vi "measure stable current with transmission.vi"(7 "na/V 2":dbl=1000.0, 8 "error in":errorcluster, 9 "measure ss":bool, 10 "field change wait(s)":u32=5, 11 "na/V":dbl=500.0) -> (0 "error out":errorcluster, 1 "stable current 2":dbl format="%.2f", 3 "stable current":dbl format="%.2f", 4 "inj current":dbl format="%#_6e", 5 "INJ ss ratio":dbl format="%#_6e")   [LabVIEW 2016]
uses:
  stable controls/stable cluster.ctl
  kubley/data acquisition 2009/beamline/controls/stable state combo.ctl
panel:
  in  "Charge State":dbl=3.0
  out "Waveform Graph 2":dbl[](graph)
  in  "measure transmission?":bool=TRUE
  in  "stable data in":T1={"injector current"=1.0, "offset current"=1.0, "ss inj ratio"=1.0, "ss offset ratio"=1.0, "transmission"=1.0, "2nd offset current"=1.0}
  out "stable data out":T1={"injector current"=1.0, "offset current"=1.0, "ss inj ratio"=1.0, "ss offset ratio"=1.0, "transmission"=1.0, "2nd offset current"=1.0}
  out "stable current 3":cluster{"data":dbl[]}[](graph)
  in  "inj current 4":dbl
  out "inj current 3":dbl format="%#_6e"
  in  "inj current 2":dbl
  out "step":string
  in  "measure stable":bool
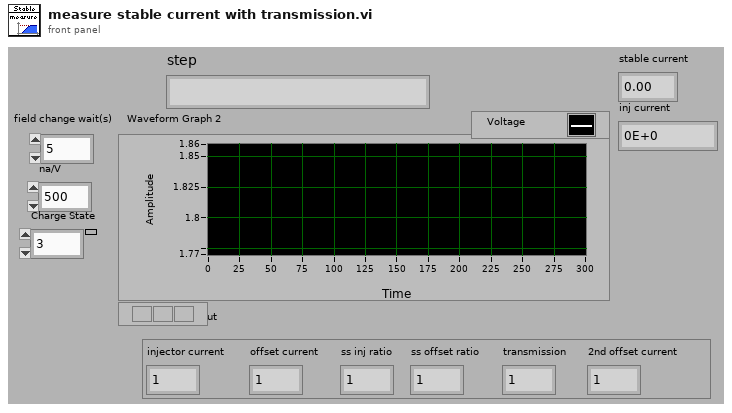
[diagram p1: front panel]
types:
  T1 = typedef "stable cluster.ctl" = cluster{"injector current":dbl, "offset current":dbl, "ss inj ratio":dbl, "ss offset ratio":dbl, "transmission":dbl, "2nd offset current":dbl}
  T2 = typedef "stable state combo.ctl" = string
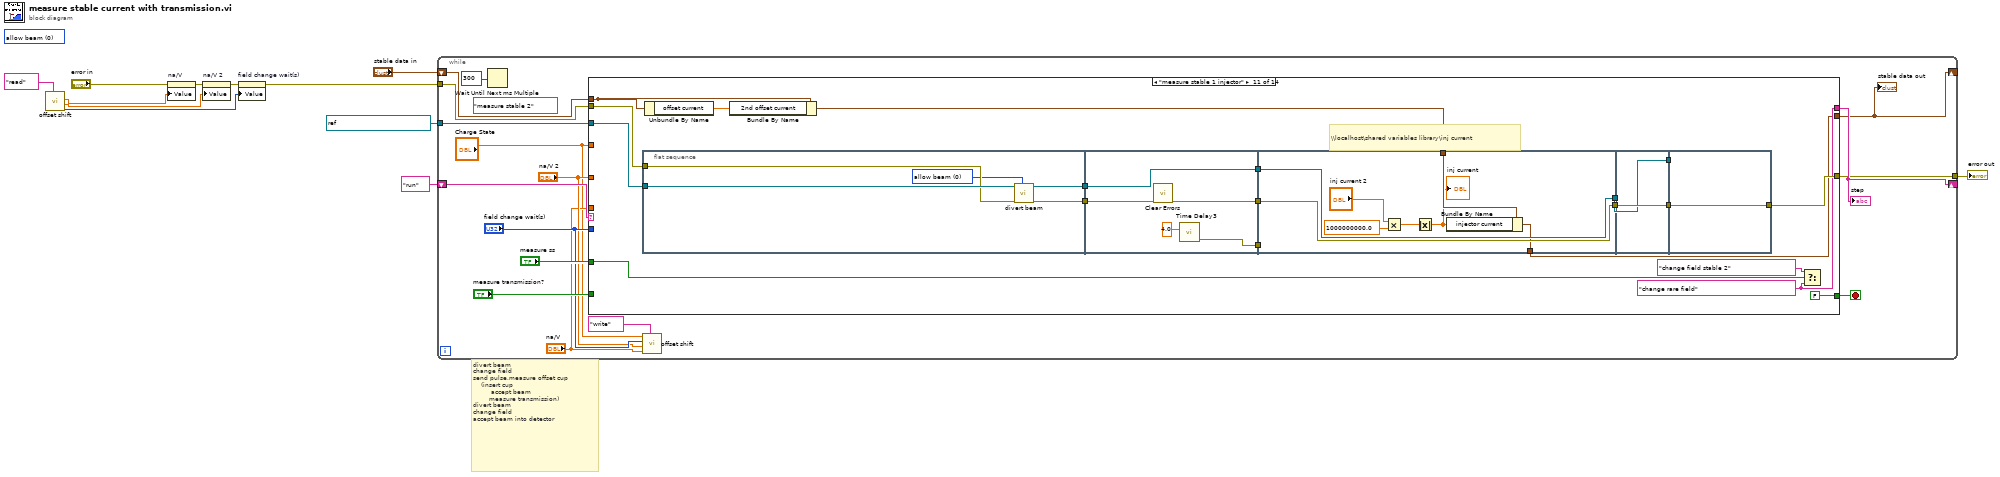
[diagram p0: block diagram]
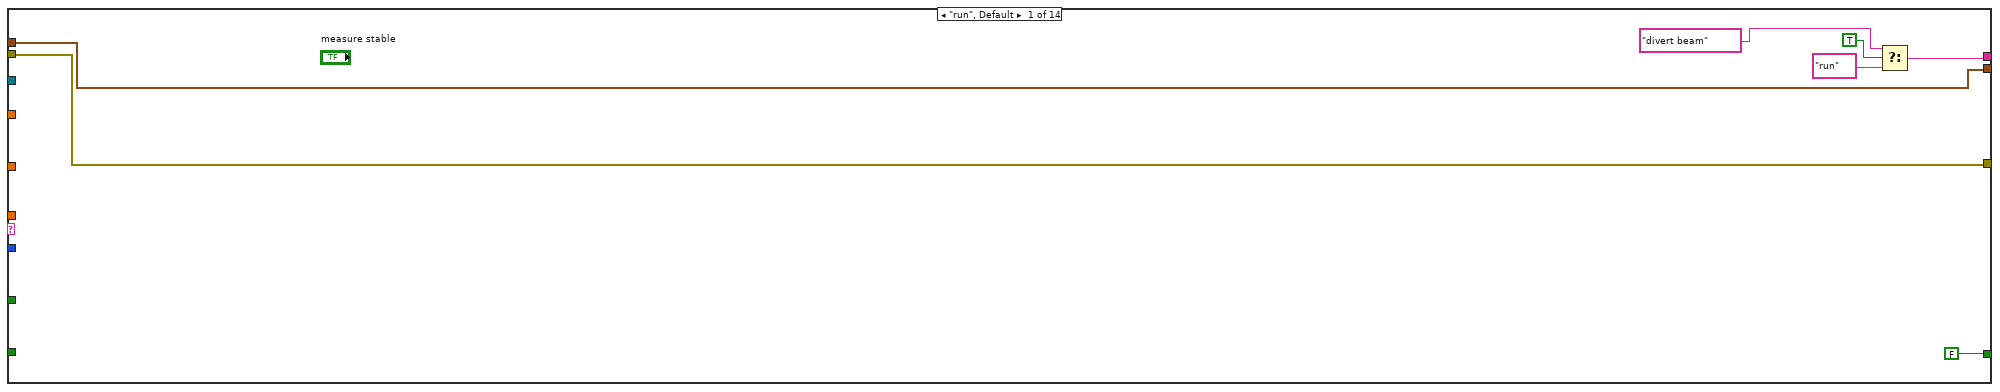
[diagram p2: hidden frame]
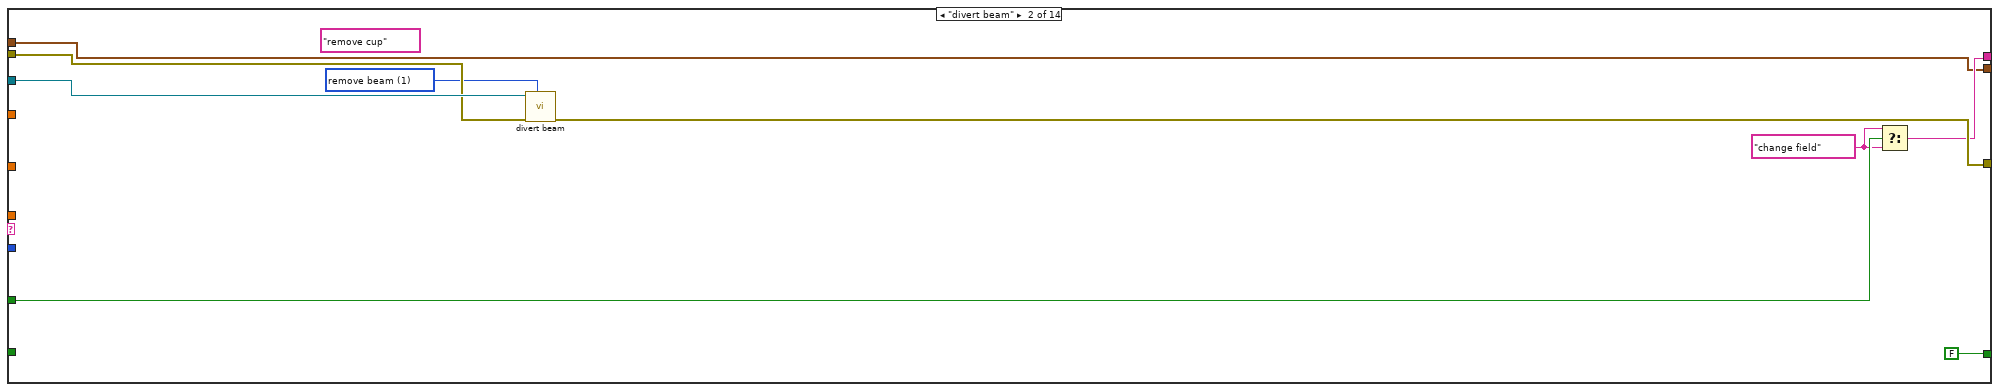
[diagram p3: hidden frame]
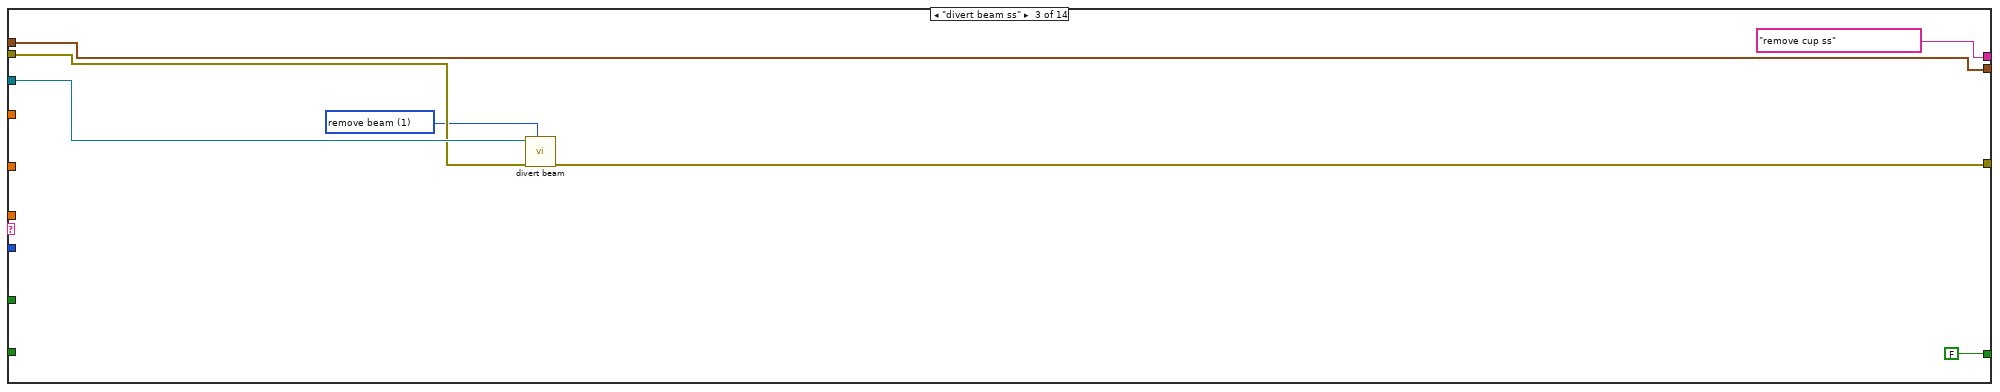
[diagram p4: hidden frame]
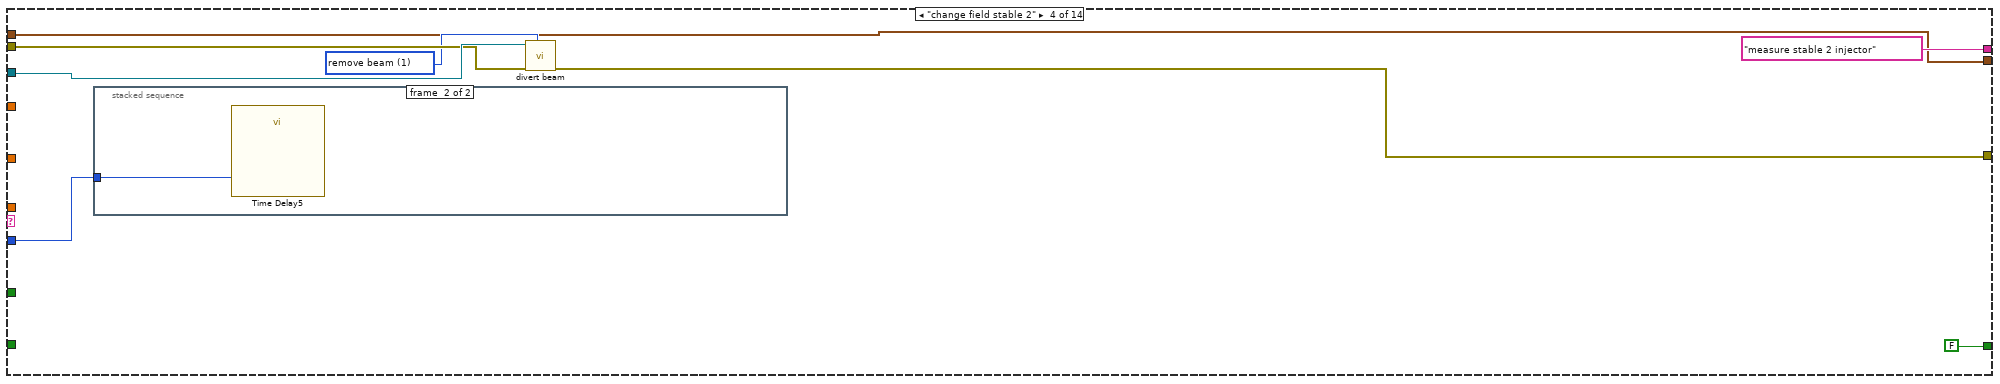
[diagram p5: hidden frame]
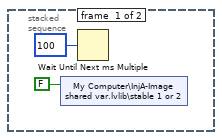
[diagram p6: hidden frame]
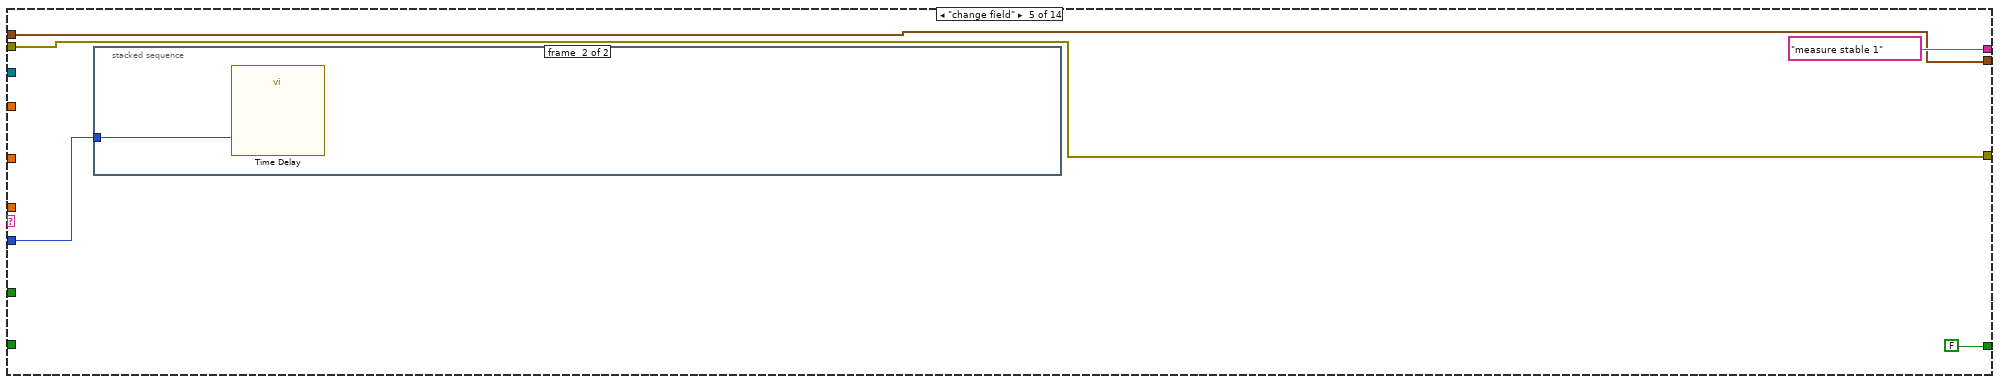
[diagram p7: hidden frame]
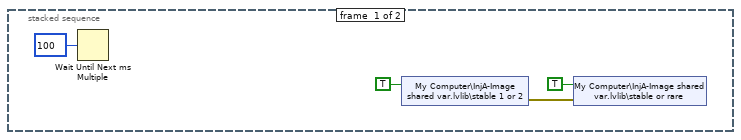
[diagram p8: hidden frame]
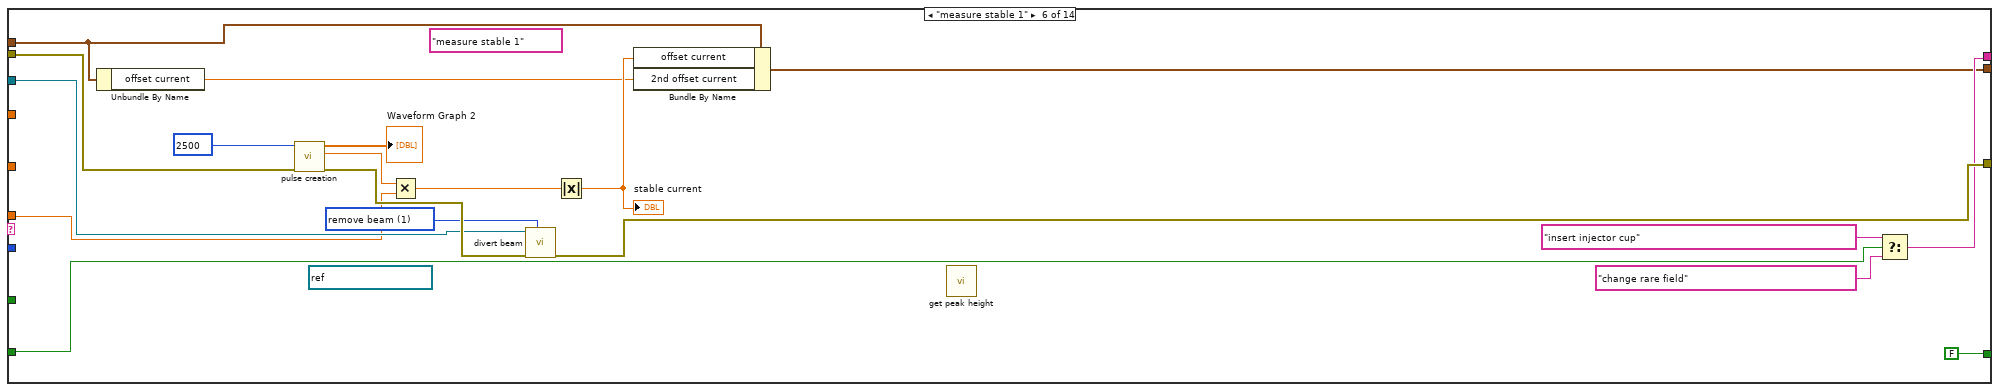
[diagram p9: hidden frame]
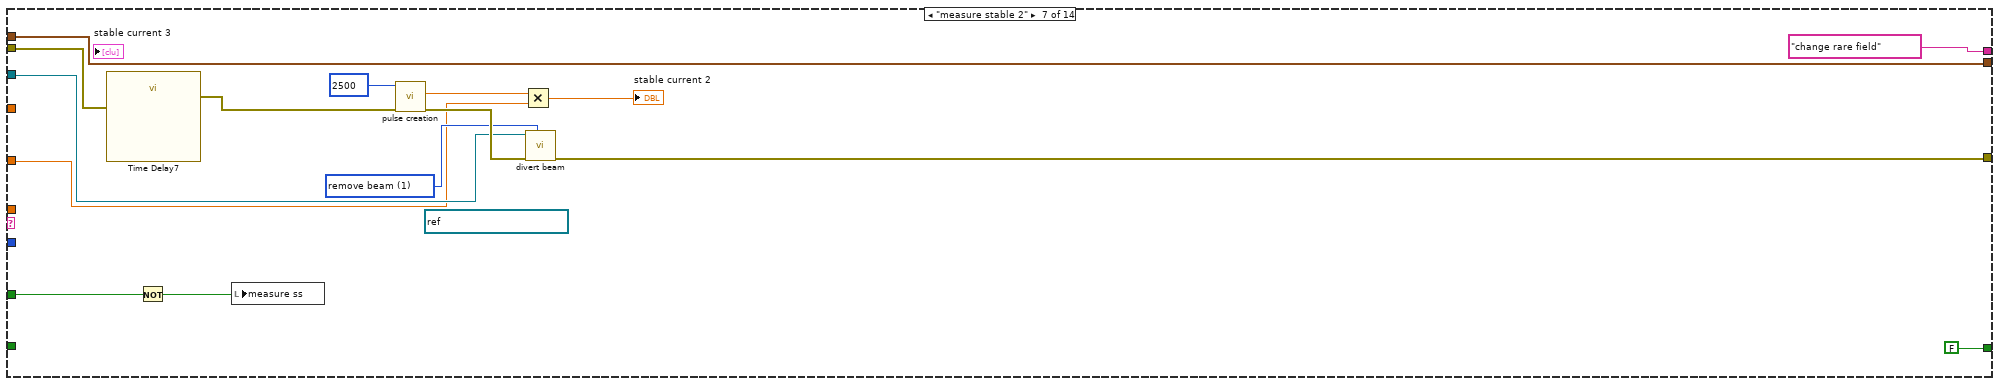
[diagram p10: hidden frame]
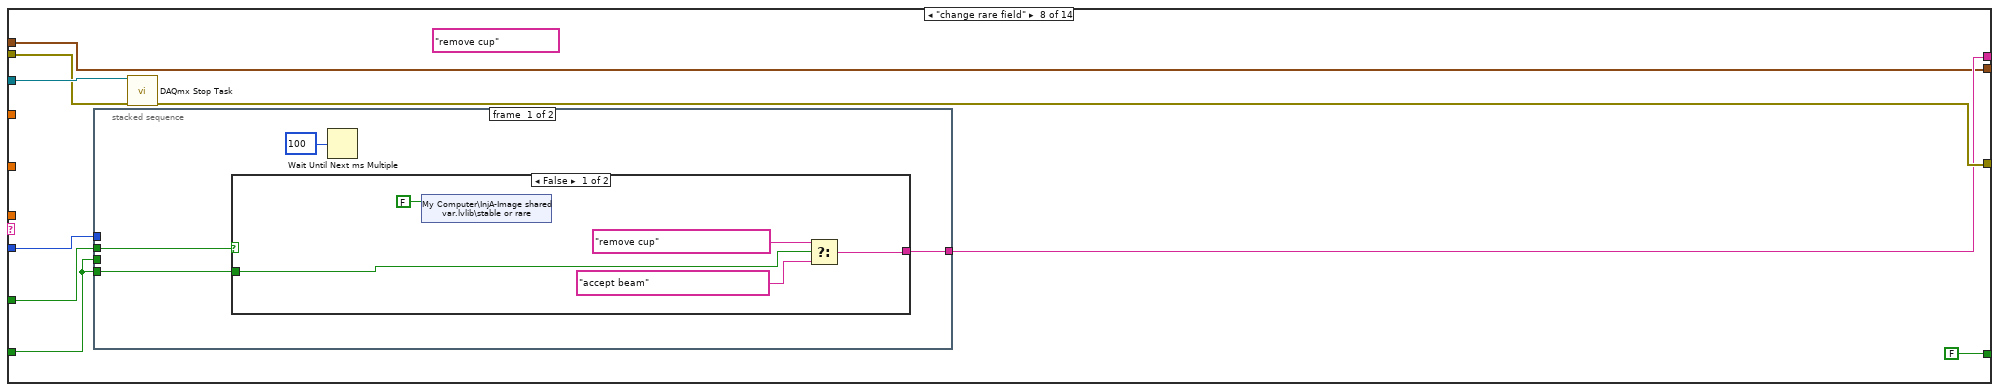
[diagram p11: hidden frame]
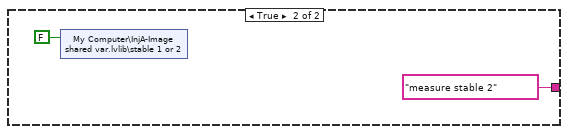
[diagram p12: hidden frame]
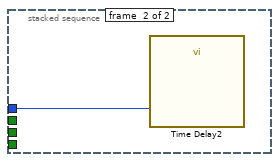
[diagram p13: hidden frame]
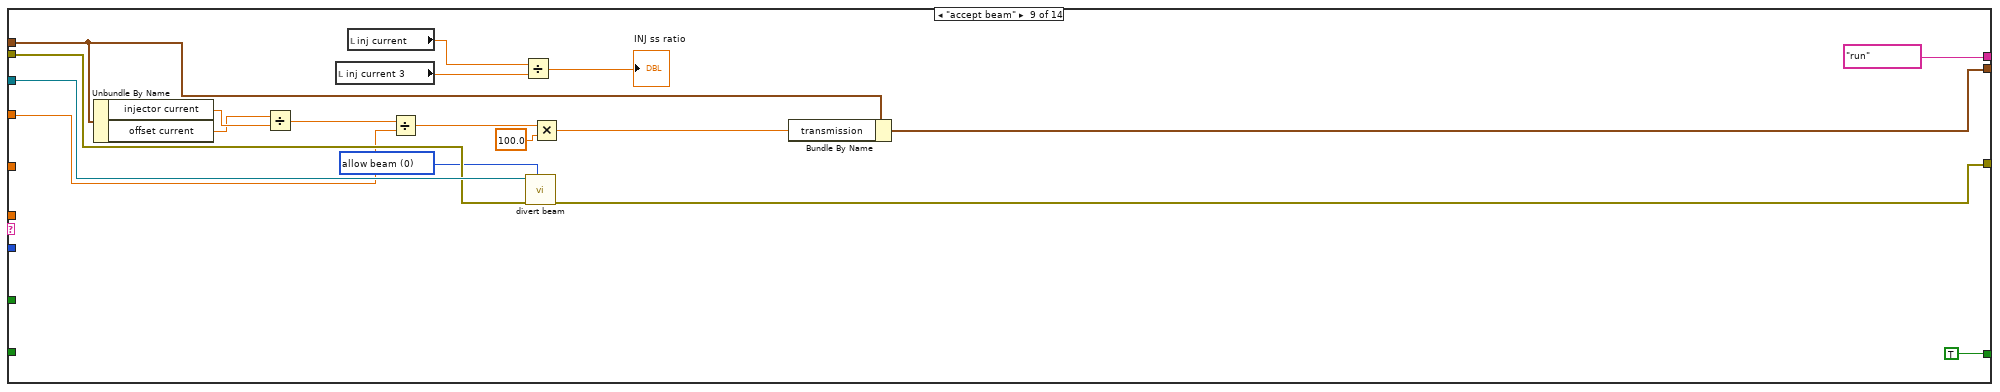
[diagram p14: hidden frame]
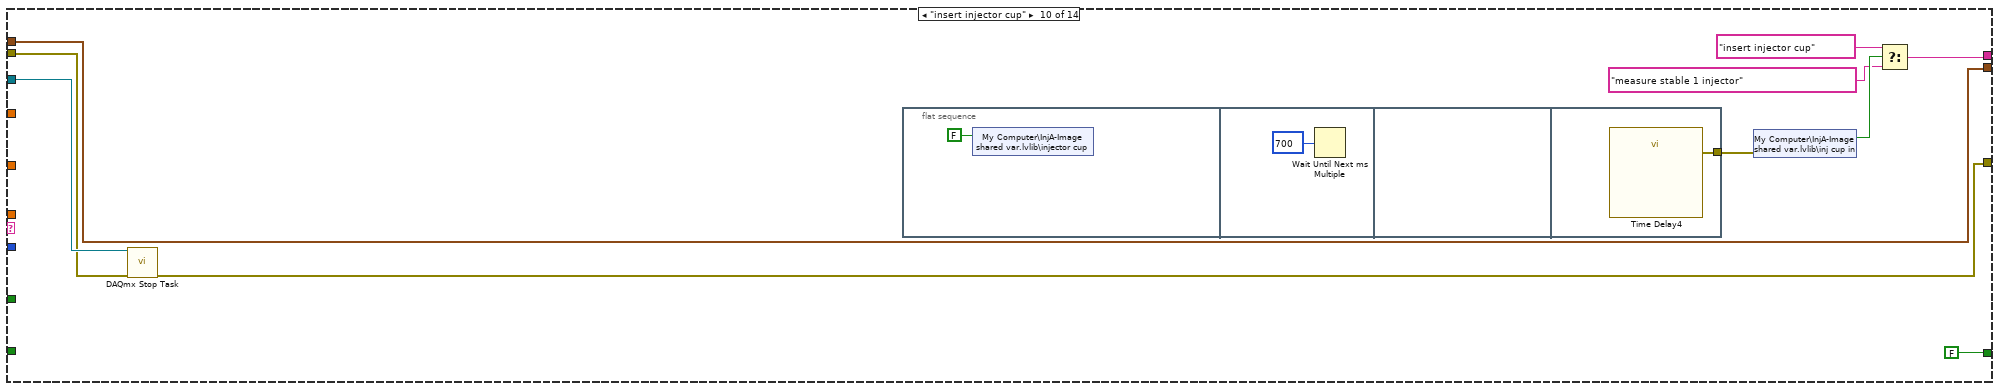
[diagram p15: hidden frame]
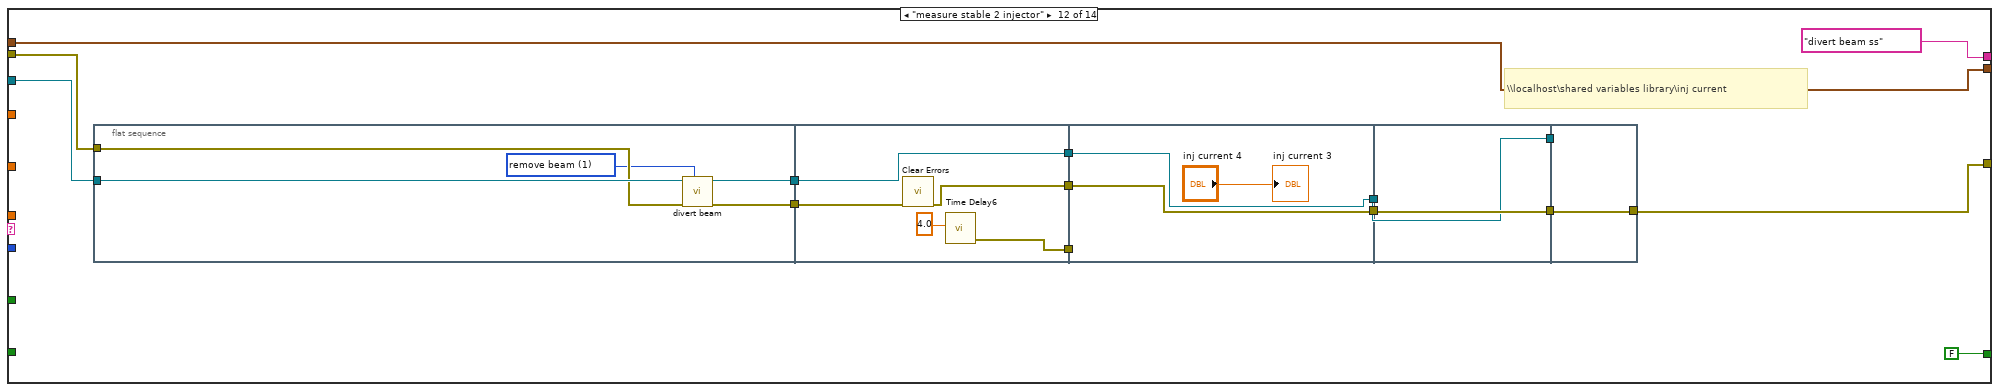
[diagram p16: hidden frame]
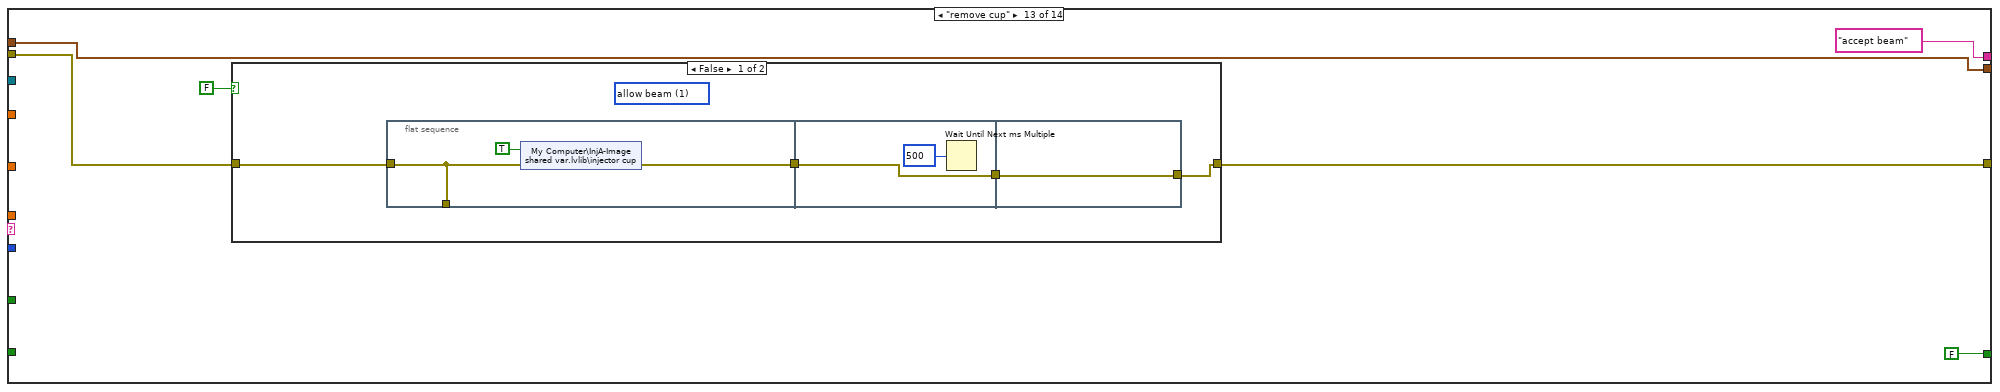
[diagram p17: hidden frame]
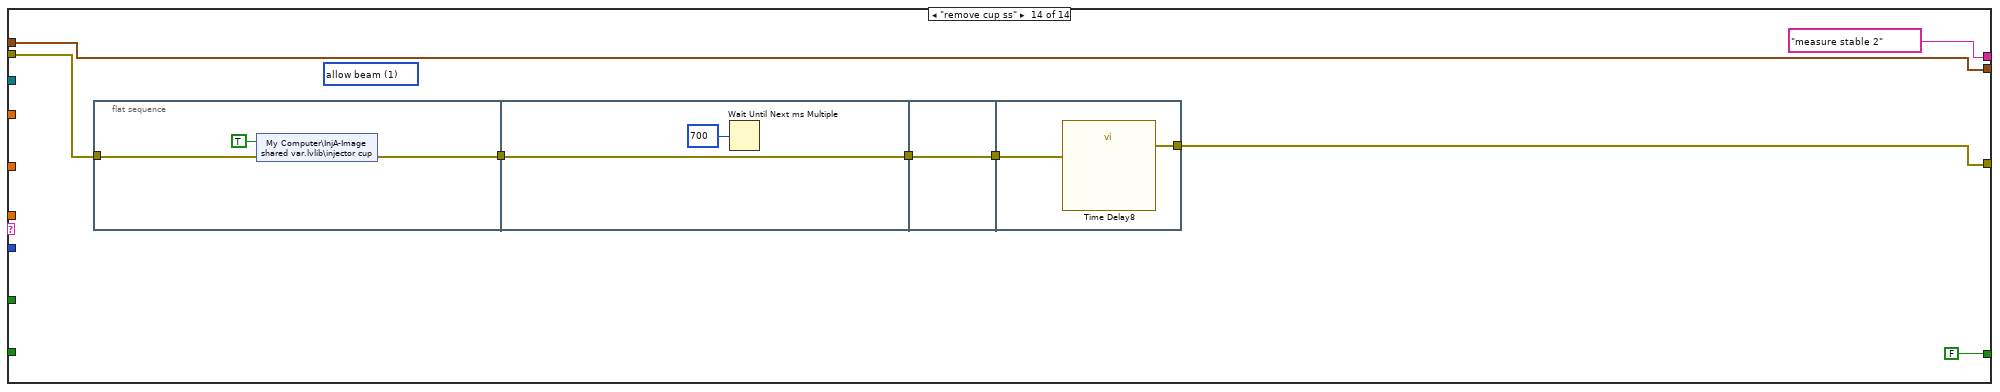
[diagram p19: hidden frame]
diagram:
  (unwired) u16 0 items=["allow beam", "remove beam"] ("divert beam? 2")
  # "divert beam\nchange field\nsend pulse,measure offset cup\n    (insert cup\n         accept beam\n        measure transmission)\ndivert beam\nchange field\naccept beam into detector"
  n1 = call "offset shift.vi"("read writ"="read") -> ("field change wait(s) out"=w8:u32, "na/V 2out"=w7:dbl, "na/V out"=w6:dbl)  [unwired: 7 in, 1 out]
  n2 = property on="na/V" class="DigNum (strict)"(error in="error in", "Value"=w6) -> (error out=w4:errorcluster)  [unwired: 1 in, 1 out]
  n3 = property on="na/V 2" class="DigNum (strict)"(error in=w4, "Value"=w7) -> (error out=w3:errorcluster)  [unwired: 1 in, 1 out]
  n4 = property on="field change wait(s)" class="DigNum (strict)"(error in=w3, "Value"=w8) -> (error out=w2:errorcluster)  [unwired: 1 in, 1 out]
  n5 = while {
    shift-right: [w27] -> _
    shift-left: T2 "run" ("stable measurement type") -> [w28]
    tunnel: refnum<k21> "stable current output" ("task/channels in") -> [w26]
    tunnel: [w24] -> w10
    tunnel: w2 -> [w23]
    shift-right: [w18] -> _
    shift-left: "stable data in" -> [w19]
    stop <- w22 stop-if-true
    (unwired) T2 "measure stable 2" ("stable measurement type")
    n6 = Wait Until Next ms Multiple(millisecond multiple=u32 300) -> ()  [unwired: 1 out]
    n7 = case shown="\"measure stable 1 injector\"" w28 {
      tunnel: [w33 w39 T2 "remove cup ss" ("stable measurement type") T2 "measure stable 2 injector" ("stable measurement type") T2 "measure stable 1" ("stable measurement type") w82 T2 "change rare field" ("stable measurement type") w108 T2 "run" ("stable measurement type") w149 w163 T2 "divert beam ss" ("stable measurement type") T2 "accept beam" ("stable measurement type") T2 "measure stable 2" ("stable measurement type")] -> w27
      tunnel: w26 -> [_ w44 w51 w59 _ w87 w103 w113 w145 w154 w175 w211 _ _]
      tunnel: "field change wait(s)" -> [_ _ _ w54 w66 _ _ w115 _ _ _ _ _ _]
      tunnel: [FALSE ("stop") FALSE ("stop") FALSE ("stop") FALSE ("stop") FALSE ("stop") FALSE ("stop") FALSE ("stop") FALSE ("stop") TRUE ("stop") FALSE ("stop") FALSE ("stop") FALSE ("stop") FALSE ("stop") FALSE ("stop")] -> w22
      tunnel: [w30 w42 w49 w56 w64 w84 w101 w111 w141 w152 w166 w202 w233 w248] -> w24
      tunnel: w23 -> [w30 w41 w48 w55 w64 w88 w97 w112 w142 w153 w172 w208 w234 w252]
      tunnel: "measure transmission?" -> [_ _ _ _ _ w86 _ w109 _ _ _ _ _ _]
      tunnel: "measure ss" -> [_ w40 _ _ _ _ w99 w110 _ _ w165 _ _ _]
      tunnel: w19 -> [w29 w36 w45 w52 w63 w76 w93 w107 w135 w148 w160 w200 w231 w253]
      tunnel: [w29 w36 w45 w52 w63 w77 w93 w107 w134 w148 w162 w200 w231 w253] -> w18
      tunnel: "Charge State" -> [_ _ _ _ _ _ _ _ w128 _ _ _ _ _]
      tunnel: "na/V" -> [_ _ _ _ _ w74 _ _ _ _ _ _ _ _]
      tunnel: "na/V 2" -> [_ _ _ _ _ _ w92 _ _ _ _ _ _ _]
      frame "run", Default {
        n8 = Select(t=T2 "divert beam" ("stable measurement type"), s=TRUE, f=T2 "run" ("stable measurement type")) -> (s? t:f=w33:T2)
      }
      frame "divert beam" {
        w37 = u16 1 items=["allow beam", "remove beam"] ("divert beam? 2")
        (unwired) T2 "remove cup" ("stable measurement type")
        w38 = T2 "change field" ("stable measurement type")
        n9 = call "divert beam.vi"("divert beam?"=w37, "error in"=w41, "task/channels in"=w44) -> ("error out"=w42:errorcluster)  [unwired: 7 in, 1 out]
        n10 = Select(t=w38, s=w40, f=w38) -> (s? t:f=w39:T2)
      }
      frame "divert beam ss" {
        w46 = u16 1 items=["allow beam", "remove beam"] ("divert beam? 2")
        n11 = call "divert beam.vi"("divert beam?"=w46, "error in"=w48, "task/channels in"=w51) -> ("error out"=w49:errorcluster)  [unwired: 7 in, 1 out]
      }
      frame "change field stable 2" {
        w53 = u16 1 items=["allow beam", "remove beam"] ("divert beam? 2")
        n12 = stacked-sequence {
          tunnel: w54 -> [_ w62]
          frame #0 {
            n13 = shared-variable "My Computer\\InjA-Image shared var.lvlib\\stable 1 or 2"(FALSE ("stable or rare")) -> ()  [unwired: 1 in, 1 out]
            n14 = Wait Until Next ms Multiple(millisecond multiple=u32 100) -> ()  [unwired: 1 out]
          }
          frame #1 {
            n15 = call "Time Delay5"("Delay Time (s)"=w62) -> ()  [unwired: 10 in, 1 out]
          }
        }
        n16 = call "divert beam.vi"("divert beam?"=w53, "error in"=w55, "task/channels in"=w59) -> ("error out"=w56:errorcluster)  [unwired: 7 in, 1 out]
      }
      frame "change field" {
        n17 = stacked-sequence {
          tunnel: w66 -> [_ w72]
          frame #0 {
            n18 = Wait Until Next ms Multiple(millisecond multiple=u32 100) -> ()  [unwired: 1 out]
            n19 = shared-variable "My Computer\\InjA-Image shared var.lvlib\\stable 1 or 2"(TRUE ("stable or rare")) -> (error out=w68:errorcluster)  [unwired: 1 in]
            n20 = shared-variable "My Computer\\InjA-Image shared var.lvlib\\stable or rare"(TRUE ("stable or rare"), error in=w68) -> ()  [unwired: 1 out]
          }
          frame #1 {
            n21 = call "Time Delay"("Delay Time (s)"=w72) -> ()  [unwired: 10 in, 1 out]
          }
        }
      }
      frame "measure stable 1" {
        w79 = u16 1 items=["allow beam", "remove beam"] ("divert beam? 2")
        (unwired) refnum<k21> "stable currents" ("task/channels in")
        (unwired) T2 "measure stable 1" ("stable measurement type")
        n22 = Unbundle By Name(w76) -> ("offset current"=w75:dbl)
        n23 = call "pulse creation.vi"("error in"=w88, "chopper width(usec)"=u32 2500) -> ("error out"=w90:errorcluster, "mean"=w80:dbl, "Waveform Graph 2"=→"Waveform Graph 2":dbl[])  [unwired: 5 in, 2 out]
        n24 = Multiply(x=w80, y=w74) -> (x*y=w81:dbl)
        n25 = call "divert beam.vi"("divert beam?"=w79, "error in"=w90, "task/channels in"=w87) -> ("error out"=w84:errorcluster)  [unwired: 7 in, 1 out]
        n26 = Absolute Value(x=w81) -> (abs(x)=w78:dbl)
        "stable current" <- w78
        n27 = Bundle By Name(cluster=w76, "offset current"=w78, "2nd offset current"=w75) -> (w77:T1)
        n28 = call "get peak height.vi"() -> ()  [unwired: 8 in, 4 out]
        n29 = Select(t=T2 "insert injector cup" ("stable measurement type"), s=w86, f=T2 "change rare field" ("stable measurement type")) -> (s? t:f=w82:T2)
      }
      frame "measure stable 2" {
        w94 = u16 1 items=["allow beam", "remove beam"] ("divert beam? 2")
        (unwired) refnum<k21> "secondary current" ("task/channels in")
        n30 = call "Time Delay7"("error in (no error)"=w97) -> ("error out"=w96:errorcluster)  [unwired: 10 in]
        n31 = Not(x=w99) -> (.not. x?=w98:bool)
        n32 = local write "measure ss"(w98) -> ()
        n33 = call "pulse creation.vi"("error in"=w96, "chopper width(usec)"=u32 2500) -> ("error out"=w105:errorcluster, "mean"=w95:dbl)  [unwired: 5 in, 3 out]
        n34 = Multiply(x=w95, y=w92) -> (x*y=→"stable current 2":dbl)
        n35 = call "divert beam.vi"("divert beam?"=w94, "error in"=w105, "task/channels in"=w103) -> ("error out"=w101:errorcluster)  [unwired: 7 in, 1 out]
      }
      frame "change rare field" {
        (unwired) T2 "remove cup" ("stable measurement type")
        n36 = stacked-sequence {
          tunnel: w115 -> [_ w127]
          tunnel: w110 -> [w118 _]
          tunnel: w109 -> [w117 _]
          tunnel: w109 -> [_ _]
          tunnel: [w116 _] -> w108
          frame #0 {
            n37 = case shown="False" w118 {
              tunnel: w117 -> [w121 _]
              tunnel: [w120 T2 "measure stable 2" ("stable measurement type")] -> w116
              frame False {
                n38 = shared-variable "My Computer\\InjA-Image shared var.lvlib\\stable or rare"(FALSE ("stable or rare")) -> ()  [unwired: 1 in, 1 out]
                n39 = Select(t=T2 "remove cup" ("stable measurement type"), s=w121, f=T2 "accept beam" ("stable measurement type")) -> (s? t:f=w120:T2)
              }
              frame True {
                n40 = shared-variable "My Computer\\InjA-Image shared var.lvlib\\stable 1 or 2"(FALSE ("stable or rare")) -> ()  [unwired: 1 in, 1 out]
              }
            }
            n41 = Wait Until Next ms Multiple(millisecond multiple=u32 100) -> ()  [unwired: 1 out]
          }
          frame #1 {
            n42 = call "Time Delay2"("Delay Time (s)"=w127) -> ()  [unwired: 10 in, 1 out]
          }
        }
        n43 = call <vilib>:"DAQmx Stop Task.vi"("task/channels in"=w113, "error in"=w112) -> ("error out"=w111:errorcluster)  [unwired: 12 in, 1 out]
      }
      frame "accept beam" {
        w137 = u16 0 items=["allow beam", "remove beam"] ("divert beam? 2")
        n44 = Unbundle By Name(w135) -> ("injector current"=w133:dbl, "offset current"=w132:dbl)
        n45 = Divide(x=w132, y=w133) -> (x/y=w136:dbl)
        n46 = local read "inj current 3"() -> (w139:dbl)
        n47 = local read "inj current"() -> (w140:dbl)
        n48 = Divide(x=w136, y=w128) -> (x/y=w131:dbl)
        n49 = Divide(x=w140, y=w139) -> (x/y=→"INJ ss ratio":dbl)
        n50 = call "divert beam.vi"("divert beam?"=w137, "error in"=w142, "task/channels in"=w145) -> ("error out"=w141:errorcluster)  [unwired: 7 in, 1 out]
        n51 = Multiply(x=w131, y=100.0) -> (x*y=w129:dbl)
        n52 = Bundle By Name(cluster=w135, "transmission"=w129) -> (w134:T1)
      }
      frame "insert injector cup" {
        n53 = call <vilib>:"DAQmx Stop Task.vi"("task/channels in"=w154, "error in"=w153) -> ("error out"=w152:errorcluster)  [unwired: 12 in, 1 out]
        n54 = flat-sequence {
          tunnel: [w158] -> w151
          frame #0 {
            n55 = shared-variable "My Computer\\InjA-Image shared var.lvlib\\injector cup"(FALSE ("injector cup")) -> ()  [unwired: 1 in, 1 out]
          }
          frame #1 {
            n56 = Wait Until Next ms Multiple(millisecond multiple=u32 700) -> ()  [unwired: 1 out]
          }
          frame #2 {
          }
          frame #3 {
            n57 = call "Time Delay4"() -> ("error out"=w158:errorcluster)  [unwired: 11 in]
          }
        }
        n58 = shared-variable "My Computer\\InjA-Image shared var.lvlib\\inj cup in"(error in=w151) -> (w150:bool)  [unwired: 1 out]
        n59 = Select(t=T2 "insert injector cup" ("f"), s=w150, f=T2 "measure stable 1 injector" ("stable measurement type")) -> (s? t:f=w149:T2)
      }
      frame "measure stable 1 injector" {
        w163 = T2 "change rare field" ("stable measurement type")
        # "\\\\localhost\\shared variables library\\inj current"
        n60 = flat-sequence {
          tunnel: w175 -> [w183]
          tunnel: [w182] -> w176
          tunnel: [w180] -> w173
          tunnel: w172 -> [w181]
          tunnel: [w186] -> w177
          tunnel: w176 -> [w187]
          tunnel: [w188] -> w174
          tunnel: w173 -> [w188]
          tunnel: [w184] -> w167
          tunnel: [w196] -> w171
          tunnel: w177 -> [w196]
          tunnel: [w195] -> w169
          tunnel: w174 -> [w195]
          tunnel: w167 -> [_]
          tunnel: w159 -> [w194]
          tunnel: [w193] -> w162
          tunnel: w171 -> [w198]
          tunnel: [w198] -> w170
          tunnel: w169 -> [w197]
          tunnel: [w197] -> w168
          tunnel: w170 -> [w199]
          tunnel: w168 -> [_]
          tunnel: [w199] -> w166
          frame #0 {
            w179 = u16 0 items=["allow beam", "remove beam"] ("divert beam? 2")
            n61 = call "divert beam.vi"("divert beam?"=w179, "error in"=w181, "task/channels in"=w183) -> ("error out"=w182:errorcluster, "task out"=w180:refnum<k21>)  [unwired: 7 in]
          }
          frame #1 {
            n62 = call <vilib>:"Clear Errors.vi"("error in (no error)"=w187) -> ("error out"=w186:errorcluster)  [unwired: 5 in, 1 out]
            n63 = call "Time Delay3"("Delay Time (s)"=4.0) -> ("error out"=w184:errorcluster)  [unwired: 10 in]
          }
          frame #2 {
            n64 = Multiply(x="inj current 2", y=1000000000.0) -> (x*y=w190:dbl)
            n65 = Absolute Value(x=w190) -> (abs(x)=w189:dbl)
            "inj current" <- w189
            n66 = Bundle By Name(cluster=w194, "injector current"=w189) -> (w193:T1)
          }
          frame #3 {
          }
          frame #4 {
          }
        }
        n67 = Unbundle By Name(w160) -> ("offset current"=w161:dbl)
        n68 = Bundle By Name(cluster=w160, "2nd offset current"=w161) -> (w159:T1)
        n69 = Select(t=T2 "change field stable 2" ("stable measurement type"), s=w165, f=w163) -> ()  [unwired: 1 out]
      }
      frame "measure stable 2 injector" {
        # "\\\\localhost\\shared variables library\\inj current"
        n70 = flat-sequence {
          tunnel: w211 -> [w219]
          tunnel: [w218] -> w212
          tunnel: [w216] -> w209
          tunnel: w208 -> [w217]
          tunnel: [w222] -> w213
          tunnel: w212 -> [w223]
          tunnel: [w224] -> w210
          tunnel: w209 -> [w224]
          tunnel: [w220] -> w203
          tunnel: [w227] -> w207
          tunnel: w213 -> [w227]
          tunnel: [w226] -> w205
          tunnel: w210 -> [w226]
          tunnel: w203 -> [_]
          tunnel: w207 -> [w229]
          tunnel: [w229] -> w206
          tunnel: w205 -> [w228]
          tunnel: [w228] -> w204
          tunnel: w206 -> [w230]
          tunnel: w204 -> [_]
          tunnel: [w230] -> w202
          frame #0 {
            w215 = u16 1 items=["allow beam", "remove beam"] ("divert beam? 2")
            n71 = call "divert beam.vi"("divert beam?"=w215, "error in"=w217, "task/channels in"=w219) -> ("error out"=w218:errorcluster, "task out"=w216:refnum<k21>)  [unwired: 7 in]
          }
          frame #1 {
            n72 = call <vilib>:"Clear Errors.vi"("error in (no error)"=w223) -> ("error out"=w222:errorcluster)  [unwired: 5 in, 1 out]
            n73 = call "Time Delay6"("Delay Time (s)"=4.0) -> ("error out"=w220:errorcluster)  [unwired: 10 in]
          }
          frame #2 {
            "inj current 3" <- "inj current 4"
          }
          frame #3 {
          }
          frame #4 {
          }
        }
      }
      frame "remove cup" {
        n74 = case shown="False" FALSE {
          tunnel: w234 -> [w238 w247]
          tunnel: [w237 w247] -> w233
          frame False {
            (unwired) u16 1 items=["divert beam", "allow beam"] ("divert beam? 2")
            n75 = flat-sequence {
              tunnel: [w241] -> _
              tunnel: w238 -> [w241]
              tunnel: [w242] -> w240
              tunnel: [w244] -> w239
              tunnel: w240 -> [w244]
              tunnel: w239 -> [w246]
              tunnel: [w246] -> w237
              frame #0 {
                n76 = shared-variable "My Computer\\InjA-Image shared var.lvlib\\injector cup"(TRUE ("injector cup"), error in=w241) -> (error out=w242:errorcluster)
              }
              frame #1 {
                n77 = Wait Until Next ms Multiple(millisecond multiple=u32 500) -> ()  [unwired: 1 out]
              }
              frame #2 {
              }
            }
          }
          frame True {
          }
        }
      }
      frame "remove cup ss" {
        (unwired) u16 1 items=["divert beam", "allow beam"] ("divert beam? 2")
        n78 = flat-sequence {
          tunnel: w252 -> [w257]
          tunnel: [w256] -> w249
          tunnel: [w259] -> w250
          tunnel: w249 -> [w259]
          tunnel: [w261] -> w251
          tunnel: w250 -> [w261]
          tunnel: [w263] -> w248
          tunnel: w251 -> [w262]
          frame #0 {
            n79 = shared-variable "My Computer\\InjA-Image shared var.lvlib\\injector cup"(TRUE ("injector cup"), error in=w257) -> (error out=w256:errorcluster)
          }
          frame #1 {
            n80 = Wait Until Next ms Multiple(millisecond multiple=u32 700) -> ()  [unwired: 1 out]
          }
          frame #2 {
          }
          frame #3 {
            n81 = call "Time Delay8"("error in (no error)"=w262) -> ("error out"=w263:errorcluster)  [unwired: 10 in]
          }
        }
      }
    }
    "step" <- w27
    "stable data out" <- w18
    n82 = call "offset shift.vi"("read writ"="write", "na/V"="na/V", "na/V 2"="na/V 2", "field change wait(s)"="field change wait(s)", "charge state"="Charge State") -> ()  [unwired: 3 in, 4 out]
  }
  "error out" <- w10
